vi "Send status.vi"(8 "error in (no error)":errorcluster, 11 "Channel in":refnum<class "Channel.lvclass">) -> (0 "error out":errorcluster, 3 "Channel out":refnum<class "Channel.lvclass">)   [LabVIEW 2018, in "Channel.lvclass"]
uses:
  Channel.lvclass
  Channel.lvclass/Channel.ctl
  Server/Server.lvclass/Server.ctl
  Simulated_CCD_Camera/Simulated Camera.lvclass/Simulated Camera.ctl
  RxTx/RxTx.lvclass
  Simulated_CCD_Camera/Simulated Camera.lvclass
  Server/Server.lvclass
panel:
  in  "comm status":T1
  in  "Prev SET parameters":T2
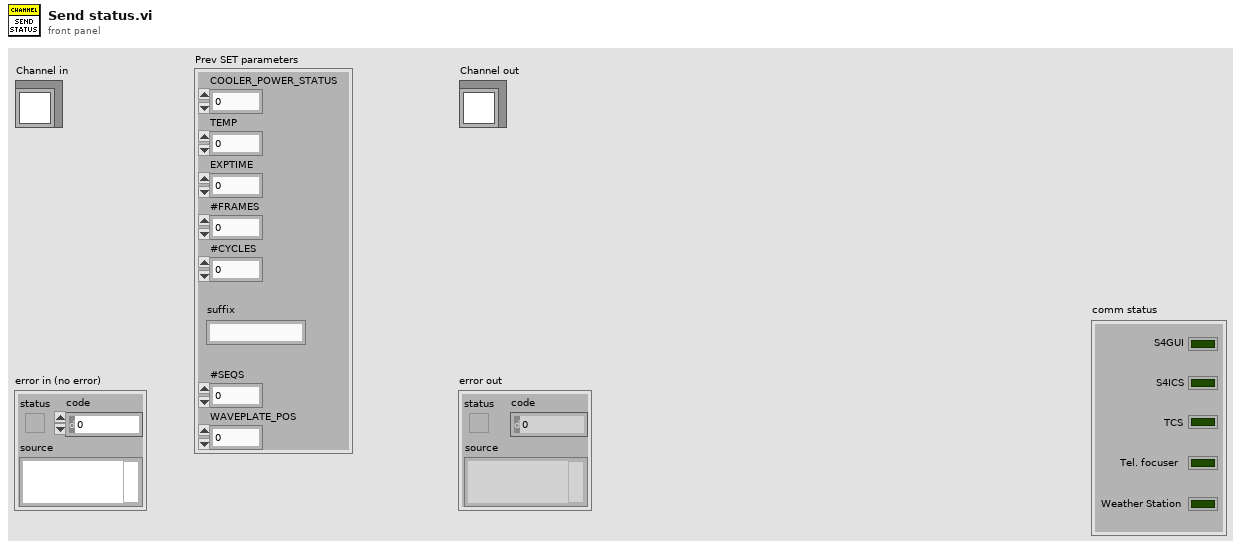
[diagram p1: front panel]
types:
  T1 = cluster{"S4GUI":bool, "S4ICS":bool, "TCS":bool, "Weather Station":bool, "Tel. focuser":bool}
  T2 = cluster{"COOLER_POWER_STATUS":u16, "TEMP":i32, "EXPTIME":dbl, "#FRAMES":u32, "#CYCLES":u32, "#SEQS":u32, "WAVEPLATE_POS":u16, "suffix":string}
  T3 = cluster{"CYCLES_DONE":u16, "LAST_IMAGE_NAME":string, "USED_DISK_SPACE":u16, "FRAMES_DONE":u16, "CCD_STATUS":string, "CURRENT_TEMPERATURE":i16, "TEMPERATURE_STATUS":string, "FRAME_EXPOSURE_TIME":sgl, "ERROR":bool, "SERIAL_NUMBER":u16, "ACQUIRING":bool, "IMAGE_INDEX":u32, "SEQS_DONE":u16}
  T4 = cluster{"PREAMP":u16, "READOUT_RATE":u16, "EM_GAIN":u16, "VERTICAL_SHIFT_SPEED":u16, "READ_MODE":u16, "FRAME_TRANSFER":bool, "VERTICAL_CLOCK_VOLTAGE":u16, "ACQUISITION_MODE":u16, "AD_CHANNEL":u16, "EM_MODE":u16, "SHUTTER_TTL":u16, "SHUTTER_OPENING_TIME":u16, "SHUTTER_CLOSING_TIME":u16, "SHUTTER_MODE":u16, "TRIGGER_MODE":u16, "VBIN":u16, "INITIAL_LINE":u16, "INITIAL_COLUMN":u16, "FINAL_LINE":u16, "FINAL_COLUMN":u16, "HBIN":u16}
  T5 = cluster{"COOLER_POWER_STATUS":u16, "TEMP":i32, "EXPTIME":dbl, "#FRAMES":u32, "#CYCLES":u32, "#SEQS":u32, "WAVEPLATE_POS":u16}
  T6 = cluster{"EXPTIME":errorcluster, "#FRAMES":errorcluster, "#CYCLES":errorcluster, "WAVEPLATE_POS":errorcluster, "TEMP":errorcluster, "COOLER_POWER_STATUS":errorcluster, "SUFFIX":errorcluster}
  T7 = cluster{"CCD status":string, "CCD configuration":string, "Acquisition configuration":string, "S4GUI JSON string":string, "WRITE SETUP error":string, "Execution error":string, "SET error":string, "Communication status":string}
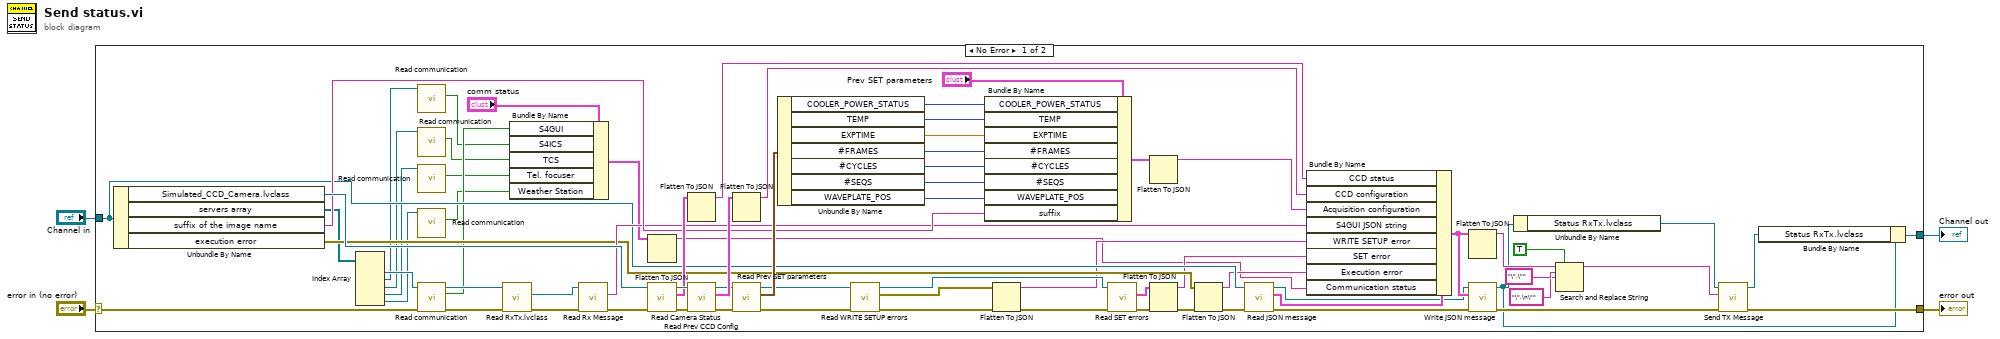
[diagram p0: block diagram]
diagram:
  n1 = case shown="No Error" "error in (no error)" {
    selector: "error in (no error)" -> [w47 w78]
    tunnel: [w74 w78] -> w3
    tunnel: [w73 w77] -> w1
    tunnel: "Channel in" -> [w41 w77]
    frame No Error {
      n2 = Unbundle By Name(w41) -> ("Simulated_CCD_Camera.lvclass"=w69:refnum<class "Simulated Camera.lvclass">, "servers array"=w5:refnum<class "Server.lvclass">[], "suffix of the image name"=w48:string, "execution error"=w29:errorcluster)
      n3 = Index Array(array=w5) -> (element #1=w21:refnum<class "Server.lvclass">, element #2=w18:refnum<class "Server.lvclass">, element #3=w17:refnum<class "Server.lvclass">, element #4=w16:refnum<class "Server.lvclass">, element #5=w15:refnum<class "Server.lvclass">)  [unwired: 5 in]
      n4 = call "Read communication.vi"("Server in"=w18) -> ("communication"=w12:bool)  [unwired: 8 in, 2 out]
      n5 = call "Read communication.vi"("Server in"=w17) -> ("communication"=w11:bool)  [unwired: 8 in, 2 out]
      n6 = call "Read communication.vi"("Server in"=w16) -> ("communication"=w10:bool)  [unwired: 8 in, 2 out]
      n7 = call "Read communication.vi"("Server in"=w15) -> ("communication"=w9:bool)  [unwired: 8 in, 2 out]
      n8 = call "Read communication.vi"("error in (no error)"=w47, "Server in"=w21) -> ("error out"=w19:errorcluster, "communication"=w13:bool, "Server out"=w20:refnum<class "Server.lvclass">)  [unwired: 7 in]
      n9 = call "Read RxTx.lvclass.vi"("error in (no error)"=w19, "Server in"=w20) -> ("error out"=w45:errorcluster, "RxTx.lvclass"=w46:refnum<class "RxTx.lvclass">)  [unwired: 7 in, 1 out]
      n10 = Bundle By Name(cluster="comm status", "S4GUI"=w13, "S4ICS"=w12, "TCS"=w11, "Tel. focuser"=w10, "Weather Station"=w9) -> (w8:T1)
      n11 = call "Read Rx Message.vi"("error in (no error)"=w45, "RxTx in"=w46) -> ("error out"=w44:errorcluster, "Rx Message"=w43:string)  [unwired: 7 in, 1 out]
      n12 = Flatten To JSON(anything=w8) -> (JSON string=w7:string)  [unwired: 2 in, 1 out]
      n13 = call "Read Camera Status.vi"("error in (no error)"=w44, "CCDCamera in"=w69) -> ("error out"=w68:errorcluster, "Camera Status"=w66:T3, "CCDCamera out"=w70:refnum<class "Simulated Camera.lvclass">)  [unwired: 7 in]
      n14 = Flatten To JSON(anything=w66) -> (JSON string=w67:string)  [unwired: 2 in, 1 out]
      n15 = call-dynamic "Read Prev CCD Config.vi"("error in (no error)"=w68, "Simulated_CCD_Camera in"=w70) -> ("error out"=w64:errorcluster, "Prev CCD Config"=w71:T4, "Simulated_CCD_Camera out"=w65:refnum<class "Simulated Camera.lvclass">)  [unwired: 7 in]
      n16 = Flatten To JSON(anything=w71) -> (JSON string=w72:string)  [unwired: 2 in, 1 out]
      n17 = call-dynamic "Read Prev SET parameters.vi"("error in (no error)"=w64, "Simulated_CCD_Camera in"=w65) -> ("error out"=w35:errorcluster, "Prev SET parameters"=w56:T5, "Simulated_CCD_Camera out"=w33:refnum<class "Simulated Camera.lvclass">)  [unwired: 7 in]
      n18 = Unbundle By Name(w56) -> ("COOLER_POWER_STATUS"=w55:u16, "TEMP"=w54:i32, "EXPTIME"=w53:dbl, "#FRAMES"=w52:u32, "#CYCLES"=w51:u32, "#SEQS"=w50:u32, "WAVEPLATE_POS"=w49:u16)
      n19 = call "Read WRITE SETUP errors.vi"("error in (no error)"=w35, "Simulated_CCD_Camera in"=w33) -> ("error out"=w25:errorcluster, "WRITE SETUP errors"=w28:errorcluster[], "Simulated_CCD_Camera out"=w34:refnum<class "Simulated Camera.lvclass">)  [unwired: 7 in]
      n20 = Bundle By Name(cluster="Prev SET parameters", "COOLER_POWER_STATUS"=w55, "TEMP"=w54, "EXPTIME"=w53, "#FRAMES"=w52, "#CYCLES"=w51, "#SEQS"=w50, "WAVEPLATE_POS"=w49, "suffix"=w48) -> (w57:T2)
      n21 = Flatten To JSON(anything=w28, error in (no error)=w25) -> (JSON string=w26:string, 11:w24:errorcluster)  [unwired: 1 in]
      n22 = call-dynamic "Read SET errors.vi"("error in (no error)"=w24, "Simulated Camera in"=w34) -> ("error out"=w32:errorcluster, "SET errors"=w23:T6)  [unwired: 7 in, 1 out]
      n23 = Flatten To JSON(anything=w57) -> (JSON string=w63:string)  [unwired: 2 in, 1 out]
      n24 = Flatten To JSON(anything=w23, error in (no error)=w32) -> (JSON string=w27:string, 11:w31:errorcluster)  [unwired: 1 in]
      n25 = Flatten To JSON(anything=w29, error in (no error)=w31) -> (JSON string=w22:string, 11:w30:errorcluster)  [unwired: 1 in]
      n26 = call-dynamic "Read JSON message.vi"("error in (no error)"=w30, "Channel in"=w41) -> ("error out"=w38:errorcluster, "JSON message"=w42:T7, "Channel out"=w39:refnum<class "Channel.lvclass">)  [unwired: 7 in]
      n27 = Bundle By Name(cluster=w42, "CCD status"=w67, "CCD configuration"=w72, "Acquisition configuration"=w63, "S4GUI JSON string"=w43, "WRITE SETUP error"=w26, "SET error"=w27, "Execution error"=w22, "Communication status"=w7) -> (w40:T7)
      n28 = Flatten To JSON(anything=w40) -> (JSON string=w62:string)  [unwired: 2 in, 1 out]
      n29 = call-dynamic "Write JSON message.vi"("error in (no error)"=w38, "JSON message"=w40, "Channel in"=w39) -> ("error out"=w37:errorcluster, "Channel out"=w36:refnum<class "Channel.lvclass">)  [unwired: 7 in]
      n30 = Unbundle By Name(w36) -> ("Status RxTx.lvclass"=w75:refnum<class "RxTx.lvclass">)
      n31 = Search and Replace String(replace all?=TRUE ("replace all? (F)"), input string=w62, search string="\",\"", replace string="\",\n\"" ("search string")) -> (result string=w6:string)  [unwired: 4 in, 3 out]
      n32 = call "Send TX Message.vi"("error in (no error)"=w37, "message"=w6, "RxTx in"=w75) -> ("error out"=w74:errorcluster, "RxTx out"=w76:refnum<class "RxTx.lvclass">)  [unwired: 7 in]
      n33 = Bundle By Name(cluster=w36, "Status RxTx.lvclass"=w76) -> (w73:refnum<class "Channel.lvclass">)
    }
    frame Error {
    }
  }
  "error out" <- w3
  "Channel out" <- w1
